vi "Write UEGO Calibration States.vi"(6 "Output Cache in":u16, 7 "UEGO Calibration States":T1, 8 "error in (no error)":errorcluster, 9 "Chip Address (A2 A1 A0)":T4 max=7, 10 "Slot #":T3 max=15, 11 "Rack #":u8) -> (0 "error out":errorcluster, 3 "FIFO SPI Message":u64 format="%b", 4 "Output Cache out":u16)   [LabVIEW 2014, in "SLSC configuration Shared.lvlib"]
doc: "Updates the FIU fault states for a single chip."
uses:
  SLSC configuration Shared.lvlib
  MCP23S17/Chip Address.ctl
  SPI Utility/Slot #.ctl
  Bank Calibration States.ctl
  Calibration State.ctl
  MCP23S17/Write Digital All Pins.vi
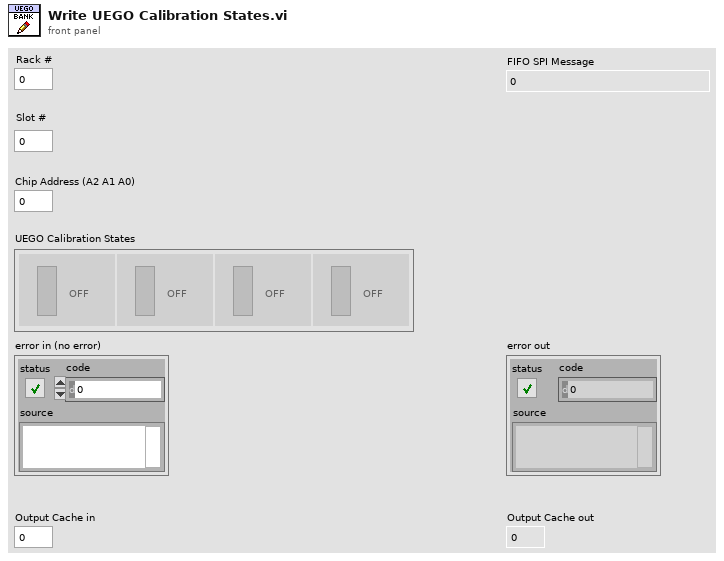
[diagram p1: front panel]
types:
  T1 = typedef "SLSC configuration Shared.lvlib/Bank Calibration States.ctl" = T2[]
  T2 = typedef "SLSC configuration Shared.lvlib/Calibration State.ctl" = bool
  T3 = typedef "SLSC configuration Shared.lvlib/Slot #.ctl" = u8
  T4 = typedef "SLSC configuration Shared.lvlib/Chip Address.ctl" = u8
  T5 = typedef "SLSC configuration Shared.lvlib/SPI Command.ctl" = cluster{"SPI Command":u32, "Transfer Length":u8}
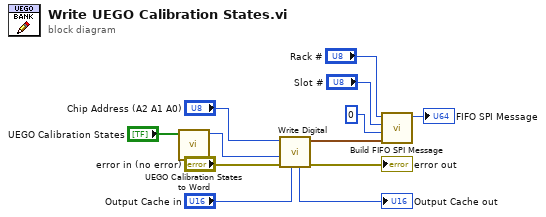
[diagram p0: block diagram]
diagram:
  n1 = call "UEGO Calibration States to Word.vi"("UEGO Calibration States"="UEGO Calibration States") -> ("UEGO Calibration Word"=w2:u16)  [unwired: 10 in]
  n2 = call-poly "Write Digital.vi"("Output Cache in"="Output Cache in", "error in (no error)"="error in (no error)", "Value"=w2, "Chip Address (A2 A1 A0)"="Chip Address (A2 A1 A0)") -> ("error out"=→"error out":errorcluster, "SPI Command"=w8:T5, "Output Cache out"=→"Output Cache out":u16)  [unwired: 5 in]
  n3 = call "Build FIFO SPI Message.vi"("SPI Command"=w8, "Chip Select"=u8 0, "Slot #"="Slot #", "Rack #"="Rack #") -> ("FIFO SPI Message"=→"FIFO SPI Message":u64)  [unwired: 7 in]
